vi "SLSC Convert EDS Property to Tree Control Item.vi"(6 "Enum string":cluster{"name":string, "enum":string}[](array[cluster]), 11 "property":T1) -> (2 "Glyph":i32, 3 "Child Text":string[](array[string]))   [LabVIEW 2015, in "SLSC Tree Control.lvlib"]
doc: "Convert the EDS property datatype to a Tree Control Child Text."
uses:
  SLSC Tree Control.lvlib
  SLSC EDS API/JSON parsing/property.ctl
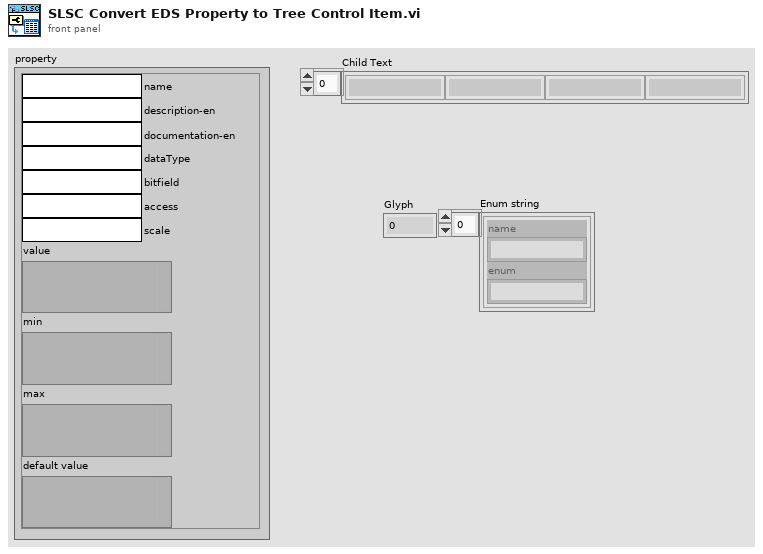
[diagram p1: front panel]
types:
  T1 = typedef "property.ctl" = cluster{"name":string, "description-en":string, "documentation-en":string, "dataType":string, "bitfield":string, "access":string, "scale":string, "value":variant, "min":variant, "max":variant, "default value":variant}
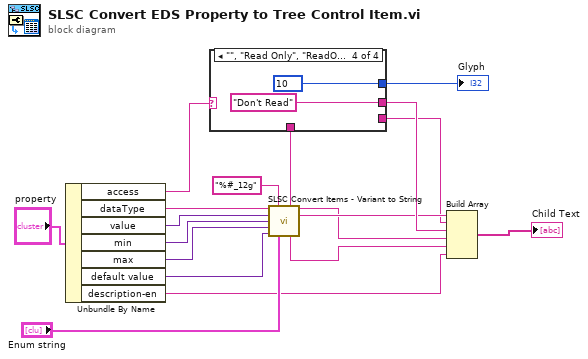
[diagram p0: block diagram]
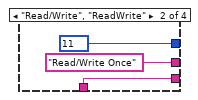
[diagram p3: hidden frame]
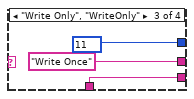
[diagram p4: hidden frame]
diagram:
  n1 = Unbundle By Name("property") -> ("access"=w12:string, "dataType"=w16:string, "value"=w15:variant, "min"=w14:variant, "max"=w10:variant, "default value"=w4:variant, "description-en"=w1:string)
  n2 = call "SLSC Convert Items - Variant to String.vi"("Datatype"=w16, "format string"="%#_12g", "value"=w15, "min"=w14, "max"=w10, "reset value"=w4, "Enum string"="Enum string") -> ("string data reset value"=w3:string, "Output data type"=w5:string, "string data value"=w6:string, "enum_range"=w7:string)  [unwired: 2 in, 3 out]
  n3 = case shown="\"\", \"Read Only\", \"ReadOnly\"" w12 {
    tunnel: [_ "Read/Write Once" ("string") "Write Once" ("string") "Don't Read" ("string")] -> w11
    tunnel: [_ 11 11 10] -> w13
    tunnel: [_ w19 w22 _] -> w2
    tunnel: w3 -> [_ w19 w22 _]
    frame Default {
    }
    frame "Read/Write", "ReadWrite" {
    }
    frame "Write Only", "WriteOnly" {
    }
    frame "", "Read Only", "ReadOnly" {
    }
  }
  "Glyph" <- w13
  n4 = Build Array(w6, w2, w11, w5, w7, w1) -> (→"Child Text":string[])
